vi "LED_Manual.vi"(8 "error in (no error)":errorcluster, 10 "Character Numeric":i32 format="%.0x", 11 "LED Notifier":refnum<notifier>) -> (0 "error out":errorcluster, 3 "LED Notifier (dup)":refnum<notifier>)   [LabVIEW 2010, in "lib1299.lvlib"]
uses:
  lib1299.lvlib
  TYP_LEDSegNotifier.ctl
  TYP_LEDCommand.ctl
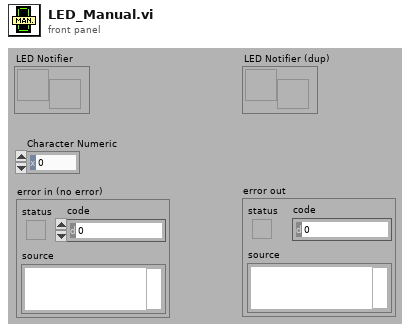
[diagram p1: front panel]
types:
  T1 = typedef "lib1299.lvlib/TYP_LEDSegNotifier.ctl" = cluster{"notification":T2, "Data":i32}
  T2 = typedef "lib1299.lvlib/TYP_LEDCommand.ctl" = enum16{"Init", "Go ACQ", "Go XFR", "Manual", "Stop", "Exit"}
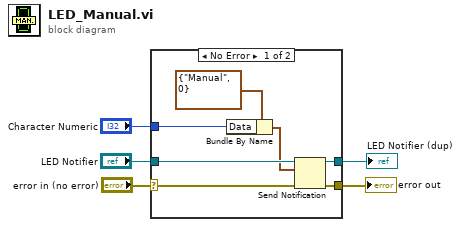
[diagram p0: block diagram]
diagram:
  n1 = case shown="No Error" "error in (no error)" {
    selector: "error in (no error)" -> [w11 w14]
    tunnel: [w12 w14] -> w5
    tunnel: "LED Notifier" -> [w10 w13]
    tunnel: "Character Numeric" -> [w7 _]
    tunnel: [w6 w13] -> w1
    frame No Error {
      n2 = Bundle By Name(cluster=T1 {"notification"=enum."Manual", "Data"=0} ("LED Display"), "Data"=w7) -> (w8:T1)
      n3 = Send Notification(notification=w8, notifier=w10, error in (no error)=w11) -> (notifier out=w6:refnum<notifier>, error out=w12:errorcluster)
    }
    frame Error {
    }
  }
  "error out" <- w5
  "LED Notifier (dup)" <- w1
